vi "BME_DG_ReserveMemory.vi"(8 "error in (no error)":errorcluster, 11 "Number of Cards":i32) -> (0 "error out":errorcluster, 3 "error code":i32)   [LabVIEW 2009]
uses:
  BME DLL/DelayGenerator.dll
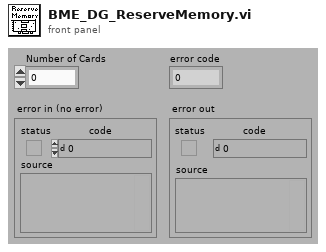
[diagram p1: front panel]
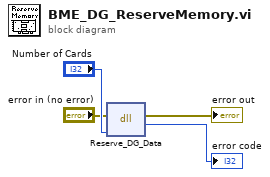
[diagram p0: block diagram]
diagram:
  n1 = dll-call lib="C:/Dokumente und Einstellungen/A2.5/Desktop/POLARIS BME DG/BME DLL/DelayGenerator.dll" fn="Reserve_DG_Data"(error in="error in (no error)", "Number of cards"="Number of Cards") -> (error out=→"error out":errorcluster, →"error code":i32)  [unwired: 3 in, 1 out]
